vi "ChangeInheritanceDialog_DEPRECATED.vi"(0 "LibWriter":refnum<class "LibWriter.lvclass">, 1 "LvClass":refnum<vi>, 5 "error in (no error)":errorcluster) -> (14 "LibWriter":refnum<class "LibWriter.lvclass">, 15 "BaseClassPath":path, 16 "Cancelled":bool, 19 "error out":errorcluster)   [LabVIEW 2014]
uses:
  <resource>/Framework/Providers/Open_GDS/ClassProviders/LibProvider_BaseClassInterface/LibWriter_class/ClassWriter_class/LibWriter.lvclass
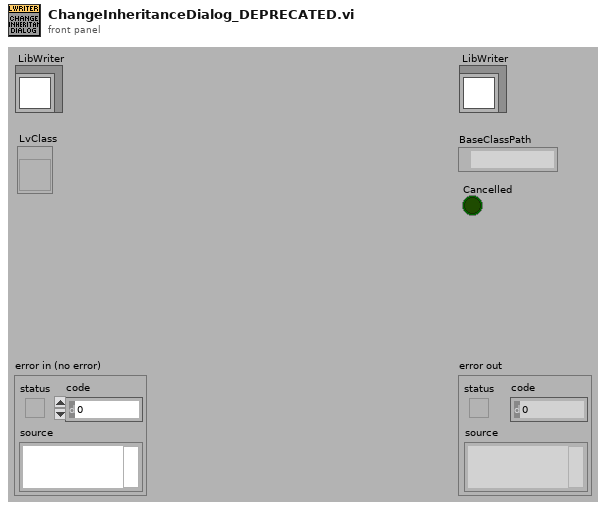
[diagram p1: front panel]
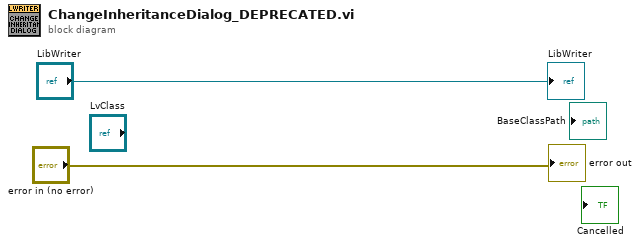
[diagram p0: block diagram]
diagram:
  "error out" <- "error in (no error)"
  "LibWriter" <- "LibWriter"
